vi "Read Screw Motor.vi"(8 "error in (no error)":errorcluster, 11 "Climber in":refnum<class "Climber.lvclass">) -> (0 "error out":errorcluster, 2 "Screw Motor":T1, 3 "Climber out":refnum<class "Climber.lvclass">)   [LabVIEW 2019, in "Climber.lvlib" / "Climber.lvclass"]
uses:
  Climber.lvclass
  Controls/Screw Motor.ctl
  Climber.lvclass/Climber.ctl
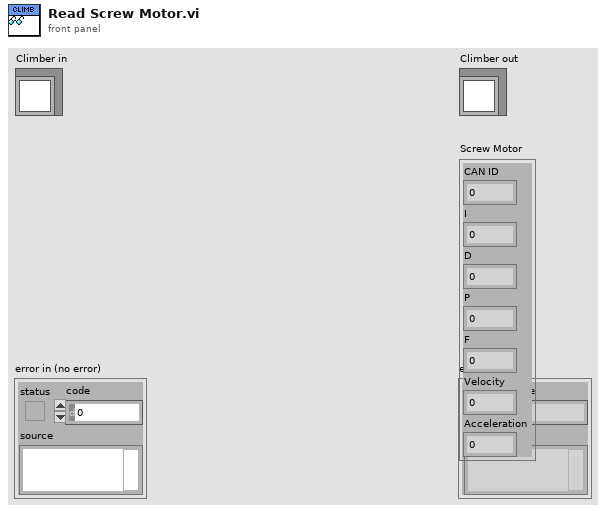
[diagram p1: front panel]
types:
  T1 = typedef "Climber.lvlib/Climber.lvclass/Screw Motor.ctl" = cluster{"CAN ID":u32, "I":dbl, "D":dbl, "P":dbl, "F":dbl, "Velocity":dbl, "Acceleration":dbl}
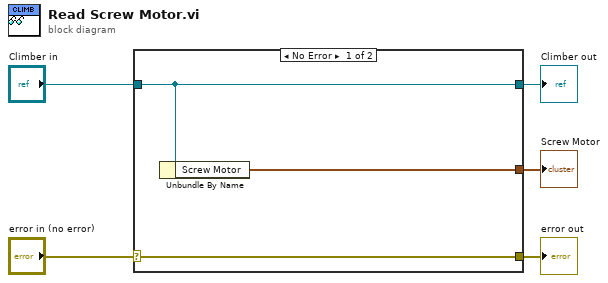
[diagram p0: block diagram]
diagram:
  n1 = case shown="No Error" "error in (no error)" {
    selector: "error in (no error)" -> [w8 w9]
    tunnel: [w8 w9] -> w4
    tunnel: [w7 w10] -> w2
    tunnel: "Climber in" -> [w7 w10]
    tunnel: [w6 _] -> w1
    frame No Error {
      n2 = Unbundle By Name(w7) -> ("Screw Motor"=w6:T1)
    }
    frame Error {
    }
  }
  "error out" <- w4
  "Climber out" <- w2
  "Screw Motor" <- w1
